vi "Do.vi"(8 "error in (no error)":errorcluster, 10 "Actor in":refnum<class "Actor.lvclass">, 11 "Set iSpkEn MSG":refnum<class "Set iSpkEn MSG.lvclass">) -> (0 "error out":errorcluster, 2 "Actor out":refnum<class "Actor.lvclass">)   [LabVIEW 2014, in "ePAS Library.lvlib" / "Set iSpkEn MSG.lvclass"]
doc: "(<B>Filename</B>: Actor Framework.lvlib:Message.lvclass:Do.vi)\n\nDefines what a message does when it is received by an actor. Generally, a message instructs an actor to invoke one of its methods. By default, this method does nothing. A child class must override it to define behavior. Create a child class by using the Actor Framework Message Maker dialog box."
uses:
  Set iSpkEn MSG.lvclass
  <vilib>/ActorFramework/Actor/Actor.lvclass
  Set iSpkEn MSG.lvclass/Set iSpkEn MSG.ctl
  Instr Actor.lvclass
  PAS/Commands/Change iSpk Signal/Change iSpk Signal.lvclass
  PAS/Commands/Change iSpk Signal/Change iSpk Signal.lvclass/Change iSpk Signal.ctl
  Controller/Messages/Update CVT/Update CVT Data.lvclass
  Controller/Messages/Update CVT/Update CVT Data.lvclass/Update CVT Data.ctl
  Controller/Messages/Update CVT/Write tag.vi
  Controller/Messages/Update CVT/Write Data.vi
  Controller/Messages/Update CVT/Write Group.vi
  PAS/Commands/Change iSpk Signal/Write iSpkEn.vi
  reusable/Command/Command.lvclass
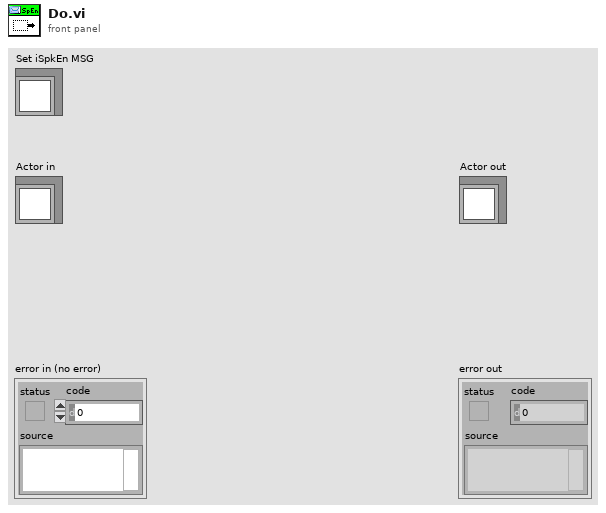
[diagram p1: front panel]
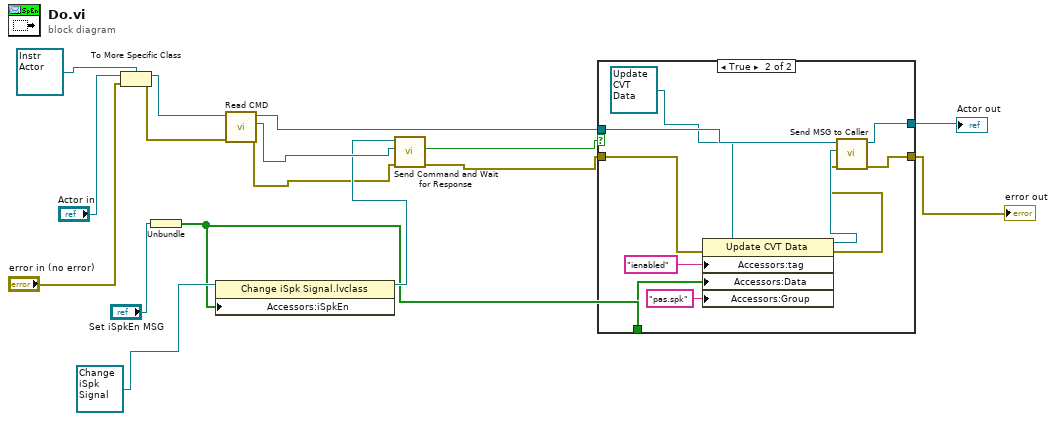
[diagram p0: block diagram]
diagram:
  n1 = To More Specific Class(target class=refnum<class "Instr Actor.lvclass"> refnum ("Instrument Lib:Instr"), reference="Actor in", error in="error in (no error)") -> (specific class reference=w14:refnum<class "Instr Actor.lvclass">, error out=w13:errorcluster)
  n2 = Unbundle("Set iSpkEn MSG") -> (w1:bool[])
  n3 = property class="Change iSpk Signal.lvclass"(reference=refnum<class "Change iSpk Signal.lvclass"> refnum ("Change iSpk Signal.lvclass"), "Accessors:iSpkEn"=w1) -> (reference out=w8:refnum<class "Change iSpk Signal.lvclass">)  [unwired: 1 in, 1 out]
  n4 = call "Read CMD.vi"("error in (no error)"=w13, "Instr Actor in"=w14) -> ("error out"=w7:errorcluster, "CMD"=w9:refnum<queue>, "Instr Actor out"=w6:refnum<class "Instr Actor.lvclass">)  [unwired: 7 in]
  n5 = call "Send Command and Wait for Response.vi"("error in"=w7, "cmd queue"=w9, "CMD in"=w8) -> ("error out"=w5:errorcluster, "cmd good?"=w4:bool)  [unwired: 6 in, 1 out]
  n6 = case shown="True" w4 {
    tunnel: w1 -> [_ w24]
    tunnel: w6 -> [w18 w28]
    tunnel: [w18 w27] -> w2
    tunnel: w5 -> [w17 w22]
    tunnel: [w17 w26] -> w3
    frame False {
    }
    frame True {
      n7 = property class="Update CVT Data"(reference=refnum<class "Update CVT Data.lvclass"> refnum ("Controller.lvlib:Update CVT Data"), error in=w22, "Accessors:tag"="ienabled" ("Key"), "Accessors:Data"=w24, "Accessors:Group"="pas.spk" ("Group")) -> (reference out=w23:refnum<class "Update CVT Data.lvclass">, error out=w21:errorcluster)
      n8 = call "Send MSG to Caller.vi"("error in"=w21, "Message"=w23, "Instr in"=w28) -> ("error out"=w26:errorcluster, "Instr out"=w27:refnum<class "Instr Actor.lvclass">)  [unwired: 7 in]
    }
  }
  "error out" <- w3
  "Actor out" <- w2
